vi "Set Marker Mode.vi"(8 "error in (no error)":errorcluster, 10 "Marker Mode (0: Sine Wave)":u32(ring) items=["Sine Wave", "Triangular / Sawtooth Pulse", "Square Wave (50 %)", "Square Wave (20 %)"], 11 "VISA resource name":refnum<visa-resource-name>) -> (0 "error out":errorcluster, 3 "VISA resource name out":refnum<visa-resource-name>)   [LabVIEW 2013, in "Fluke 5XXX Series Multicalibrators.lvlib"]
doc: "This VI selects the waveform for Marker scope mode.\n\nNote:\n\nThis VI is available only for instrument models 5500A and 5520A with oscilloscope option SC600 (SC1100)."
uses:
  Fluke 5XXX Series Multicalibrators.lvlib
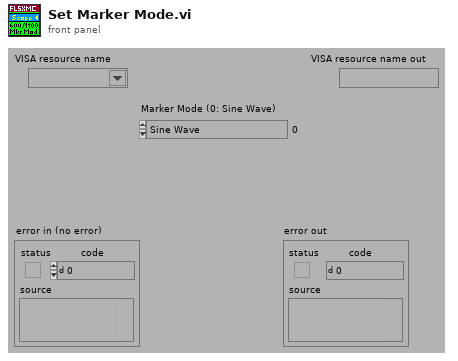
[diagram p1: front panel]
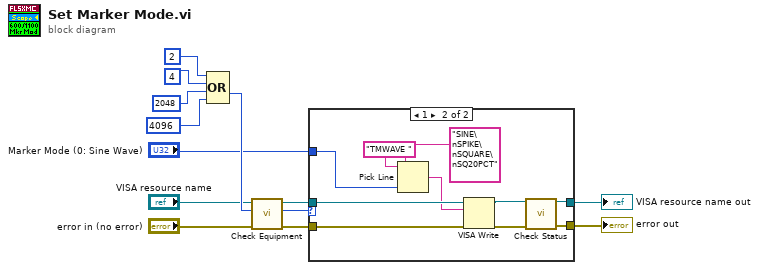
[diagram p0: block diagram]
diagram:
  n1 = Compound Arithmetic op=OR(2 ("Numeric"), 4 ("Numeric"), 2048 ("Numeric"), 4096 ("Numeric")) -> (w7:i32)
  n2 = call "Check Equipment.vi"("error in (no error)"="error in (no error)", "Bit Mask"=w7, "VISA resource name"="VISA resource name") -> ("error out"=w10:errorcluster, "Present?"=w9:u32, "VISA resource name out"=w8:refnum<visa-resource-name>)  [unwired: 6 in]
  n3 = case shown="1" w9 {
    tunnel: [w14 w17] -> w4
    tunnel: w10 -> [w15 w23]
    tunnel: w8 -> [w14 w22]
    tunnel: [w15 w20] -> w5
    tunnel: "Marker Mode (0: Sine Wave)" -> [_ w16]
    frame 0, Default {
    }
    frame 1 {
      n4 = Pick Line(string ("")="TMWAVE " ("Reset Command"), multi-line string="SINE\nSPIKE\nSQUARE\nSQ20PCT", line index=w16) -> (output string=w21:string)
      n5 = VISA Write(VISA resource name=w22, write buffer=w21, error in (no error)=w23) -> (VISA resource name out=w18:refnum<visa-resource-name>, error out=w19:errorcluster)  [unwired: 1 out]
      n6 = call "Check Status.vi"("VISA resource name"=w18, "error in (no error)"=w19) -> ("VISA resource name out"=w17:refnum<visa-resource-name>, "error out"=w20:errorcluster)  [unwired: 12 in]
    }
  }
  "VISA resource name out" <- w4
  "error out" <- w5
